vi "SeCrTs-RPM_Module_L.vi"(7 "Data FIFO Ref":T1, 8 "error in (no error)":errorcluster, 11 "TCP Network Connection in":refnum<k5>) -> (0 "error out":errorcluster, 3 "TCP Network Connection out":refnum<k5>)   [LabVIEW 2022 SP3]
uses:
  RT Controls/SeCrTs-Data FIFO.ctl
  RT Controls/SeCrTs-FGV Read write.ctl
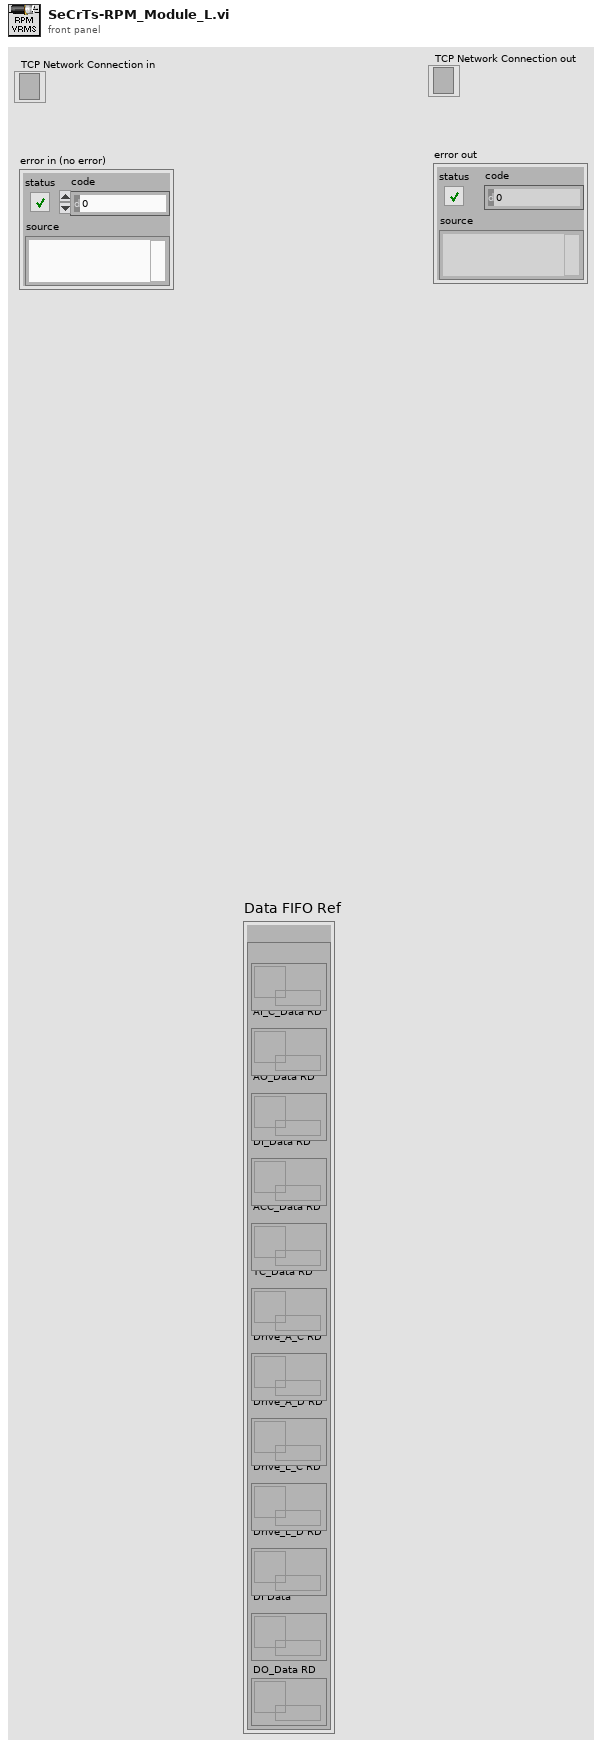
[diagram p1: front panel]
types:
  T1 = typedef "SeCrTs-Data FIFO.ctl" = cluster{"RD":cluster{"AI_V_Data RD":refnum<queue>, "AI_C_Data RD":refnum<queue>, "AO_Data RD":refnum<queue>, "DI_Data RD":refnum<queue>, "ACC_Data RD":refnum<queue>, "TC_Data RD":refnum<queue>, "Drive_A_C RD":refnum<queue>, "Drive_A_D RD":refnum<queue>, "Drive_L_C RD":refnum<queue>, "Drive_L_D RD":refnum<queue>, "DI Data":refnum<queue>, "DO_Data RD":refnum<queue>}}
  T2 = enum16{"Standard", "Buffered", "CRLF", "Immediate"}
  T3 = typedef "SeCrTs-FGV Read write.ctl" = enum16{"Write", "Read"}
  T4 = cluster{"En_Drive_A":bool, "En_Drive_L":bool, "Exit_Drive_A":bool, "Exit_Drive_L":bool}
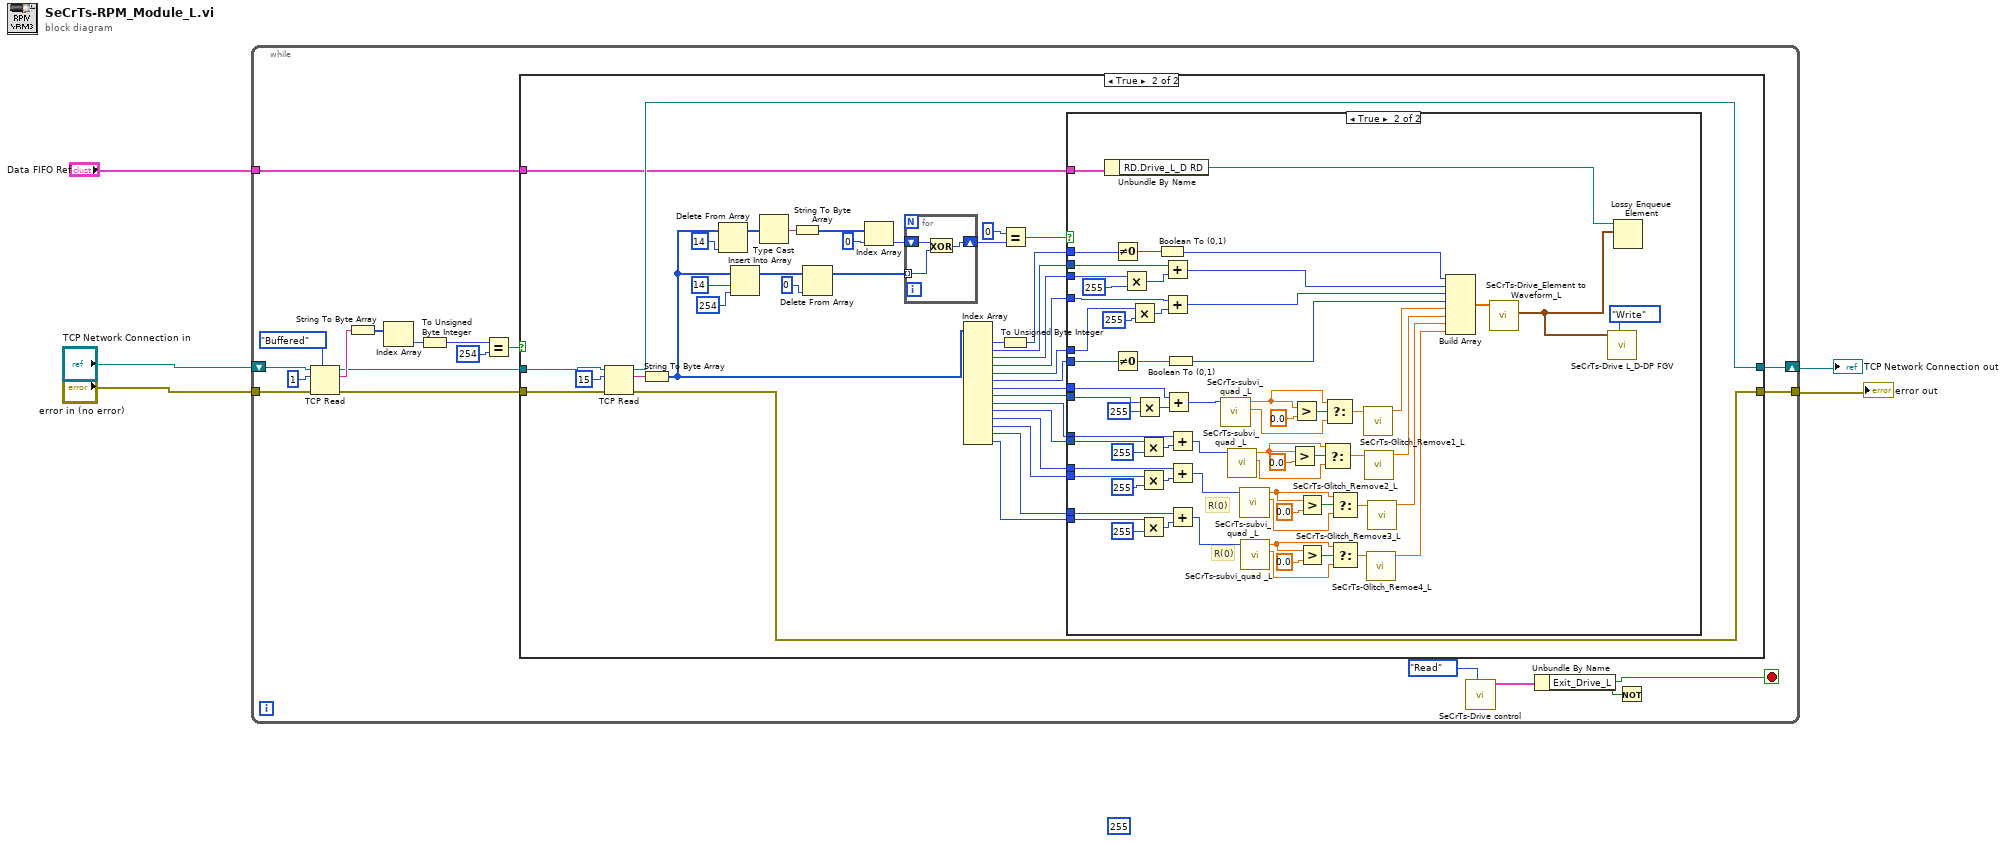
[diagram p0: block diagram]
diagram:
  (unwired) u8 255
  n1 = while {
    tunnel: "error in (no error)" -> [w22]
    shift-right: [w11] -> w5
    shift-left: "TCP Network Connection in" -> [w23]
    tunnel: [w12] -> w4
    tunnel: "Data FIFO Ref" -> [w6]
    stop <- w7 stop-if-true
    n2 = TCP Read(connection ID=w23, bytes to read=1, error in (no error)=w22, 7:T2."Buffered" ("mode (standard)")) -> (connection ID out=w15:refnum<k5>, data out=w21:string, error out=w14:errorcluster)  [unwired: 1 in]
    n3 = String To Byte Array(string=w21) -> (unsigned byte array=w20:u8[])
    n4 = Index Array(array=w20) -> (element=w19:u8)  [unwired: 1 in]
    n5 = To Unsigned Byte Integer(number=w19) -> (unsigned 8bit integer=w18:u8)
    n6 = Equal?(x=w18, y=u8 254) -> (x = y?=w16:bool)
    n7 = case shown="True" w16 {
      tunnel: w15 -> [w25 w62]
      tunnel: w14 -> [w24 w61]
      tunnel: [w25 w51] -> w11
      tunnel: [w24 w36] -> w12
      tunnel: w6 -> [_ w26]
      frame False {
      }
      frame True {
        n8 = TCP Read(connection ID=w62, bytes to read=15, error in (no error)=w61) -> (connection ID out=w51:refnum<k5>, data out=w59:string, error out=w36:errorcluster)  [unwired: 2 in]
        n9 = String To Byte Array(string=w59) -> (unsigned byte array=w44:u8[])
        n10 = Delete From Array(array=w44, index=14) -> (array with subset deleted=w57:u8[])  [unwired: 1 in, 1 out]
        n11 = Insert Into Array(array=w44, index=14, new element=u8 254 ("new element/subarray")) -> (w50:u8[])
        n12 = Type Cast(x=w57) -> (*(type *) &x=w56:string)  [unwired: 1 in]
        n13 = String To Byte Array(string=w56) -> (unsigned byte array=w55:u8[])
        n14 = Delete From Array(array=w50, index=0) -> (array with subset deleted=w47:u8[])  [unwired: 1 in, 1 out]
        n15 = Index Array(array=w55, index=0) -> (element=w48:u8)
        n16 = for {
          shift-right: [w129] -> w46
          shift-left: w48 -> [w130]
          tunnel: w47 -> [w128] mode=indexing
          n17 = Exclusive Or(1:w128, 2:w130) -> (0:w129:u8)
        }
        n18 = Index Array(array=w44) -> (element #1=w43:u8, element #2=w41:u8, element #3=w40:u8, element #4=w39:u8, element #5=w38:u8, element #6=w37:u8, element #7=w34:u8, element #8=w33:u8, element #9=w32:u8, element #10=w31:u8, element #11=w30:u8, element #12=w29:u8, element #13=w28:u8, element #14=w27:u8)  [unwired: 14 in]
        n19 = Equal?(x=u8 0, y=w46) -> (x = y?=w45:bool)
        n20 = To Unsigned Byte Integer(number=w43) -> (unsigned 8bit integer=w42:u8)
        n21 = case shown="True" w45 {
          tunnel: w42 -> [_ w127]
          tunnel: w41 -> [_ w84]
          tunnel: w40 -> [_ w83]
          tunnel: w39 -> [_ w82]
          tunnel: w38 -> [_ w81]
          tunnel: w37 -> [_ w123]
          tunnel: w34 -> [_ w114]
          tunnel: w33 -> [_ w113]
          tunnel: w32 -> [_ w112]
          tunnel: w31 -> [_ w111]
          tunnel: w30 -> [_ w110]
          tunnel: w29 -> [_ w109]
          tunnel: w28 -> [_ w108]
          tunnel: w27 -> [_ w107]
          tunnel: w26 -> [_ w66]
          frame False {
          }
          frame True {
            # "R(0)"
            # "R(0)"
            n22 = Unbundle By Name(w66) -> ("RD.Drive_L_D RD"=w65:refnum<queue>)
            n23 = Not Equal To 0?(x=w127) -> (x != 0?=w87:bool)
            n24 = Not Equal To 0?(x=w123) -> (x != 0?=w86:bool)
            n25 = Multiply(x=w83, y=u32 255) -> (x*y=w85:u32)
            n26 = Multiply(x=w81, y=u32 255) -> (x*y=w124:u32)
            n27 = Multiply(x=w113, y=u32 255) -> (x*y=w115:u32)
            n28 = Multiply(x=w111, y=u32 255) -> (x*y=w118:u32)
            n29 = Multiply(x=w109, y=u32 255) -> (x*y=w119:u32)
            n30 = Multiply(x=w107, y=u32 255) -> (x*y=w122:u32)
            n31 = Boolean To (0,1)(Boolean=w87) -> (0, 1=w76:i16)
            n32 = Add(x=w84, y=w85) -> (x+y=w75:u32)
            n33 = Add(x=w82, y=w124) -> (x+y=w74:u32)
            n34 = Add(x=w114, y=w115) -> (x+y=w80:u32)
            n35 = Boolean To (0,1)(Boolean=w86) -> (0, 1=w73:i16)
            n36 = Add(x=w112, y=w118) -> (x+y=w79:u32)
            n37 = Add(x=w110, y=w119) -> (x+y=w78:u32)
            n38 = Add(x=w108, y=w122) -> (x+y=w77:u32)
            n39 = call "SeCrTs-subvi_quad _L.vi"("input variable"=w80) -> ("output variable 2"=w97:dbl, "output variable"=w98:dbl)  [unwired: 8 in]
            n40 = call "SeCrTs-subvi_quad _L.vi"("input variable"=w79) -> ("output variable 2"=w95:dbl, "output variable"=w96:dbl)  [unwired: 8 in]
            n41 = call "SeCrTs-subvi_quad _L.vi"("input variable"=w78) -> ("output variable 2"=w93:dbl, "output variable"=w94:dbl)  [unwired: 8 in]
            n42 = call "SeCrTs-subvi_quad _L.vi"("input variable"=w77) -> ("output variable 2"=w91:dbl, "output variable"=w92:dbl)  [unwired: 8 in]
            n43 = Greater?(x=w96, y=0.0) -> (0:w101:bool)
            n44 = Greater?(x=w98, y=0.0) -> (0:w99:bool)
            n45 = Greater?(x=w94, y=0.0) -> (0:w103:bool)
            n46 = Greater?(x=w92, y=0.0) -> (0:w105:bool)
            n47 = Select(t=w96, s=w101, f=w95) -> (s? t:f=w90:dbl)
            n48 = Select(t=w98, s=w99, f=w97) -> (s? t:f=w68:dbl)
            n49 = Select(t=w94, s=w103, f=w93) -> (s? t:f=w89:dbl)
            n50 = Select(t=w92, s=w105, f=w91) -> (s? t:f=w88:dbl)
            n51 = call "SeCrTs-Glitch_Remove1_L.vi"("Input"=w68) -> ("Output"=w67:dbl)  [unwired: 10 in]
            n52 = call "SeCrTs-Glitch_Remove2_L.vi"("Input"=w90) -> ("Output"=w72:dbl)  [unwired: 10 in]
            n53 = call "SeCrTs-Glitch_Remoe4_L.vi"("Input"=w88) -> ("Output"=w70:dbl)  [unwired: 10 in]
            n54 = call "SeCrTs-Glitch_Remove3_L.vi"("Input"=w89) -> ("Output"=w71:dbl)  [unwired: 10 in]
            n55 = Build Array(w76, w75, w74, w73, w67, w72, w71, w70) -> (w69:dbl[])
            n56 = call "SeCrTs-Drive_Element to Waveform_L.vi"("Array input"=w69) -> ("RPM out"=w63:waveform(dbl)[])  [unwired: 10 in]
            n57 = call "SeCrTs-Drive L_D-DP FGV.vi"("Write/Read"=SeCrTs-FGV_Read_write."Write", "Drive L_D FGV"=w63) -> ()  [unwired: 8 in, 2 out]
            n58 = Lossy Enqueue Element(queue=w65, element=w63) -> ()  [unwired: 1 in, 4 out]
          }
        }
      }
    }
    n59 = call "SeCrTs-Drive control.vi"("Action"=enum16{"Init", "Write", "Read"}."Read") -> ("Loop Control Out"=w8:T4)  [unwired: 9 in, 1 out]
    n60 = Unbundle By Name(w8) -> ("Exit_Drive_L"=w7:bool)
    n61 = Not(x=w7) -> ()  [unwired: 1 out]
  }
  "TCP Network Connection out" <- w5
  "error out" <- w4
